vi "fgt set digital Output.vi"(8 "error in (no error)":errorcluster, 9 "on/off":bool, 10 "port":u8, 11 "controllerIndex":u32) -> (0 "error out":errorcluster)   [LabVIEW 2016, in "fgt_SDK.lvlib"]
doc: "Set the digital output ON or OFF on a controller. This feature is only available on the F-OEM device.\nOn the F-OEM, port 0 is the pump control, port 1 toggles the onboard LED."
uses:
  fgt_SDK.lvlib
  dlls/fgt_SDK_32.dll
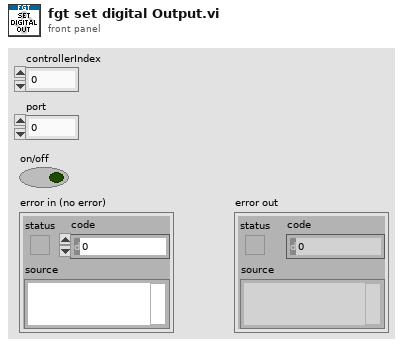
[diagram p1: front panel]
types:
  T1 = typedef "fgt_SDK.lvlib/fgt_STATUS_INFO.ctl" = cluster{"InstrType":T2, "instrSN":u16, "errorCode":u8, "infoCode":u8, "detail":string}
  T2 = typedef "fgt_SDK.lvlib/fgt_INSTRUMENT_TYPE.ctl" = enum32{"None", "MFCS", "MFCS_EZ", "FRP", "LineUP", "IPS"}
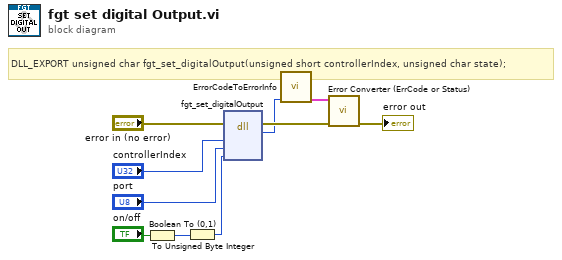
[diagram p0: block diagram]
diagram:
  # "DLL_EXPORT unsigned char fgt_set_digitalOutput(unsigned short controllerIndex, unsigned char state);"
  n1 = Boolean To (0,1)(Boolean="on/off") -> (0, 1=w3:i16)
  n2 = To Unsigned Byte Integer(number=w3) -> (unsigned 8bit integer=w2:u8)
  n3 = dll-call lib="C:/projects/SDK/fgt-sdk-labview/dlls/fgt_SDK_*.*" fn="fgt_set_digitalOutput"(error in="error in (no error)", "controllerIndex"="controllerIndex", "port"="port", "state"=w2) -> (error out=w8:errorcluster, "return type"=w6:u8)  [unwired: 5 in, 1 out]
  n4 = call "ErrorCodeToErrorInfo.vi"("return type"=w6) -> ("StatusInfo"=w5:T1)  [unwired: 10 in]
  n5 = call "Error Converter (ErrCode or Status).vi"("error in (no error)"=w8, "StatusInfo"=w5) -> ("error out"=→"error out":errorcluster)  [unwired: 9 in]
